vi "RF627_EXAMPLE_x86.vi"() -> ()   [LabVIEW 2019]
doc: "This example VI calls the .NET DLL that accompanies it, which is a .NET class built in C# to emulate a very basic calculator."
uses:
  C:/Users/aagolovachev/Desktop/RLD_T14_2dScan/src/RF62X/RF62X-SDK/examples/LabVIEW/rf62Xsdk.dll
  rf62Xsdk.dll
panel:
  in  "protocol":i32(ring)=1 items=["SERVICE_PROTOKOL"=1, "ETHERNET_IP"=2, "MODBUS_TCP"=3]
  out "Capacity":i32
  out "Connect 2":bool
  in  "?":bool
  out "Connect":bool
  out "Count Points":i32
  out "XY Graph":cluster{"X":sgl, "Z":sgl}[](graph)
  out "Count":i32
  out "SdkInit":bool
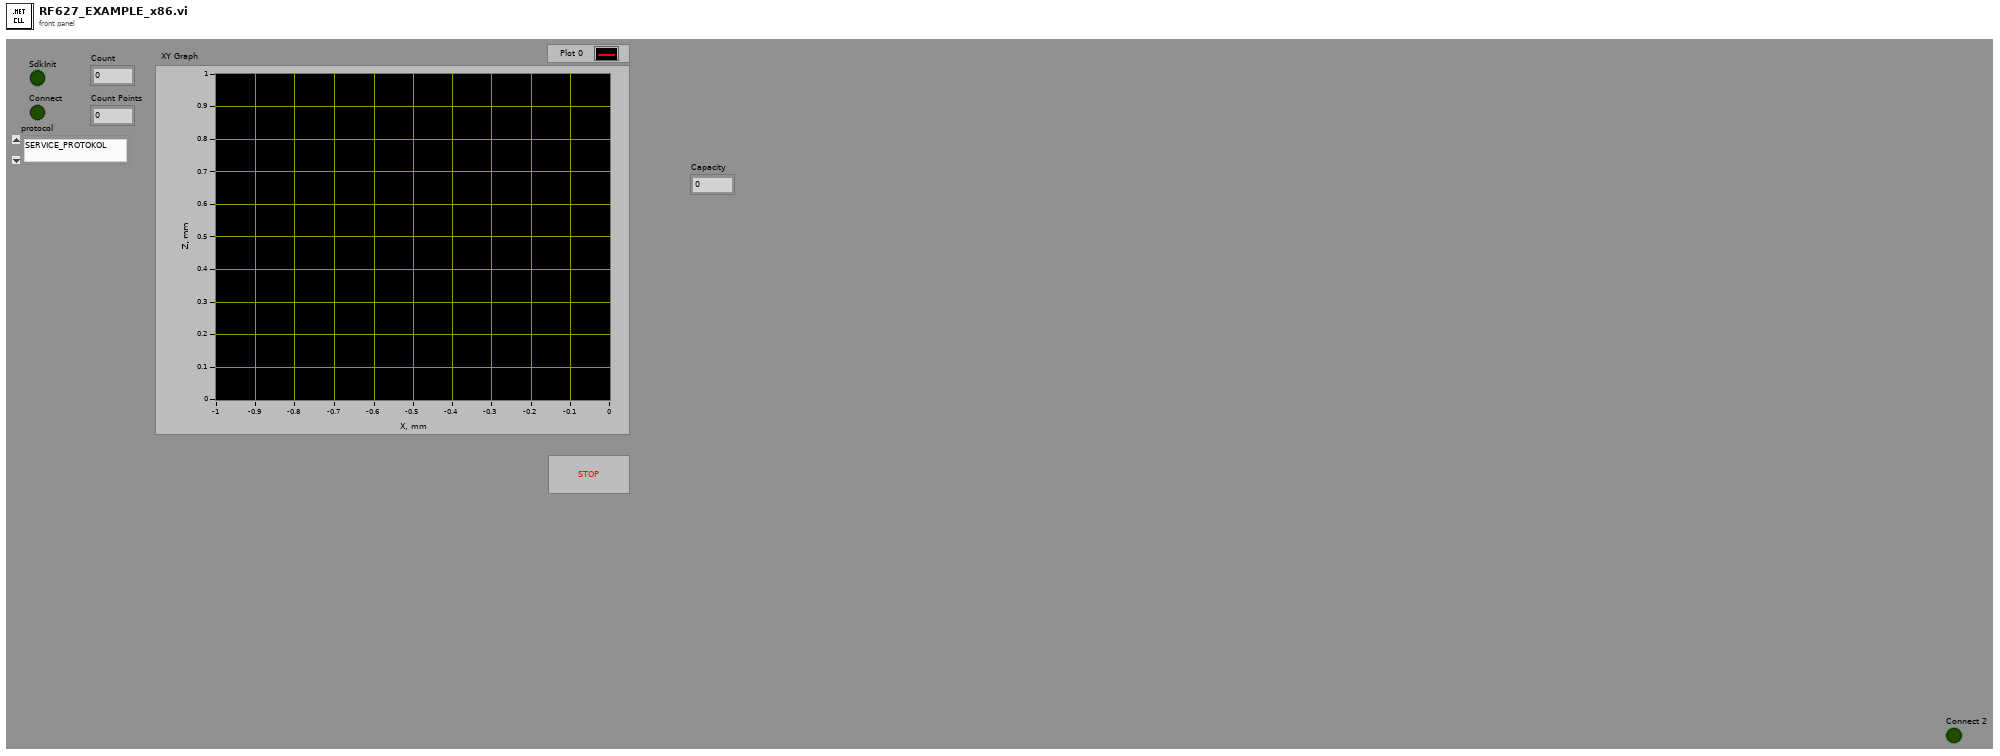
[diagram p1: front panel]
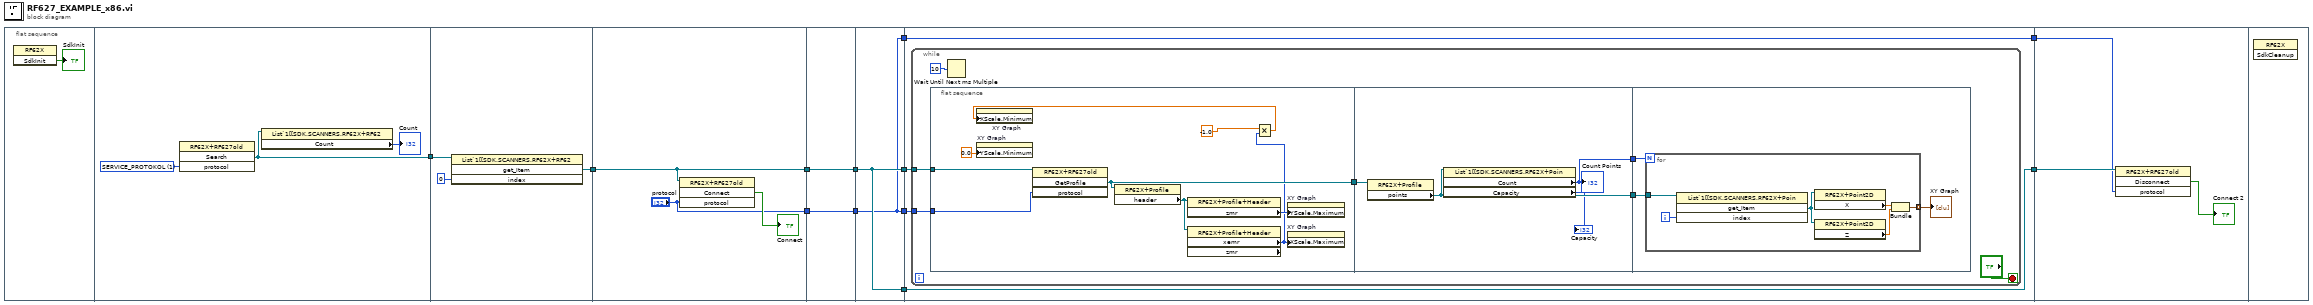
[diagram p0: block diagram]
diagram:
  n1 = flat-sequence {
    tunnel: [w14] -> w10
    tunnel: [w18] -> w12
    tunnel: w10 -> [w17]
    tunnel: w12 -> [w22]
    tunnel: [w22] -> w11
    tunnel: ["protocol"] -> w5
    tunnel: w11 -> [w24]
    tunnel: [w24] -> w8
    tunnel: w5 -> [w23]
    tunnel: [w23] -> w4
    tunnel: [w26] -> w9
    tunnel: w8 -> [w26]
    tunnel: [w26] -> w6
    tunnel: w4 -> [w25]
    tunnel: [w25] -> w3
    tunnel: [w25] -> w1
    tunnel: w9 -> [w30]
    tunnel: [w29] -> w7
    tunnel: w6 -> [w29]
    tunnel: w3 -> [w28]
    tunnel: [w27] -> w2
    tunnel: w1 -> [w27]
    tunnel: w7 -> [w61]
    tunnel: w2 -> [w60]
    frame #0 {
      n2 = invoke class="RF62X" method="SdkInit"() -> ("SdkInit"=→"SdkInit":bool)  [unwired: 3 in, 2 out]
    }
    frame #1 {
      w16 = 1 items=["SERVICE_PROTOKOL"=1, "ETHERNET_IP"=2, "MODBUS_TCP"=3] ("protocol")
      n3 = invoke class="RF62X+RF627old" method="Search"("protocol"=w16) -> ("Search"=w14:refnum<k24>)  [unwired: 3 in, 3 out]
      n4 = property class="List`1[[SDK.SCANNERS.RF62X+RF62"(reference=w14) -> ("Count"=→"Count":i32)  [unwired: 1 in, 2 out]
    }
    frame #2 {
      n5 = invoke class="List`1[[SDK.SCANNERS.RF62X+RF62" method="get_Item"(reference=w17, "index"=0) -> ("get_Item"=w18:refnum<k24>)  [unwired: 2 in, 3 out]
    }
    frame #3 {
      n6 = invoke class="RF62X+RF627old" method="Connect"(reference=w22, "protocol"="protocol") -> ("Connect"=→"Connect":bool)  [unwired: 2 in, 3 out]
    }
    frame #4 {
    }
    frame #5 {
    }
    frame #6 {
      n7 = while {
        tunnel: w30 -> [w35]
        tunnel: w28 -> [w31]
        stop <- "?" stop-if-true
        n8 = flat-sequence {
          tunnel: w35 -> [w46]
          tunnel: [w43] -> w34
          tunnel: w31 -> [w38]
          tunnel: w34 -> [w50]
          tunnel: [w49] -> w33
          tunnel: [w48] -> w32
          tunnel: w33 -> [w52]
          tunnel: w32 -> [w51]
          frame #0 {
            n9 = property on="XY Graph" class="XYGraph (strict)"("YScale.Minimum"=0.0 ("Y Scale.Range:Minimum")) -> ()  [unwired: 2 in, 2 out]
            n10 = invoke class="RF62X+RF627old" method="GetProfile"(reference=w46, "protocol"=w38) -> ("GetProfile"=w43:refnum<k24>)  [unwired: 2 in, 3 out]
            n11 = property class="RF62X+Profile"(reference=w43) -> ("header"=w44:refnum<k24>)  [unwired: 1 in, 2 out]
            n12 = property class="RF62X+Profile+Header"(reference=w44) -> ("zmr"=w45:u16)  [unwired: 1 in, 2 out]
            n13 = property class="RF62X+Profile+Header" props=["xemr", "zmr"](reference=w44) -> ("xemr"=w40:u16)  [unwired: 1 in, 3 out]
            n14 = Multiply(x=-1.0 ("Y Scale.Range:Minimum"), y=w40) -> (x*y=w39:dbl)
            n15 = property on="XY Graph" class="XYGraph (strict)"("XScale.Minimum"=w39) -> ()  [unwired: 2 in, 2 out]
            n16 = property on="XY Graph" class="XYGraph (strict)"("YScale.Maximum"=w45) -> ()  [unwired: 2 in, 2 out]
            n17 = property on="XY Graph" class="XYGraph (strict)"("XScale.Maximum"=w40) -> ()  [unwired: 2 in, 2 out]
          }
          frame #1 {
            n18 = property class="RF62X+Profile"(reference=w50) -> ("points"=w49:refnum<k24>)  [unwired: 1 in, 2 out]
            n19 = property class="List`1[[SDK.SCANNERS.RF62X+Poin"(reference=w49) -> ("Count"=w48:i32, "Capacity"=→"Capacity":i32)  [unwired: 1 in, 2 out]
            "Count Points" <- w48
          }
          frame #2 {
            n20 = for {
              N: w51 -> [_]
              tunnel: [w58] -> w53 mode=indexing
              tunnel: w52 -> [w54]
              i -> [w59]
              n21 = invoke class="List`1[[SDK.SCANNERS.RF62X+Poin" method="get_Item"(reference=w54, "index"=w59) -> ("get_Item"=w57:refnum<k24>)  [unwired: 2 in, 3 out]
              n22 = property class="RF62X+Point2D"(reference=w57) -> ("X"=w56:sgl)  [unwired: 1 in, 2 out]
              n23 = property class="RF62X+Point2D"(reference=w57) -> ("Z"=w55:sgl)  [unwired: 1 in, 2 out]
              n24 = Bundle("X"=w56, "Z"=w55) -> (w58:cluster{"X":sgl, "Z":sgl})  [unwired: 1 in]
            }
            "XY Graph" <- w53
          }
        }
        n25 = Wait Until Next ms Multiple(millisecond multiple=u32 10 ("millisecond timer value")) -> ()  [unwired: 1 out]
      }
    }
    frame #7 {
      n26 = invoke class="RF62X+RF627old" method="Disconnect"(reference=w61, "protocol"=w60) -> ("Disconnect"=→"Connect 2":bool)  [unwired: 2 in, 3 out]
    }
    frame #8 {
      n27 = invoke class="RF62X" method="SdkCleanup"() -> ()  [unwired: 3 in, 3 out]
    }
  }
